vi "Midterm2.vi"() -> ()   [LabVIEW 2019]
uses:
  Program Files (x86)/National Instruments/LabVIEW 2019/project/EN1Course-master (12)/EN1Course-master/_Subs/ThingWorx/_TW_Subs/TW_XControl.xctl
  Program Files (x86)/National Instruments/LabVIEW 2019/project/EN1Course-master (12)/EN1Course-master/_Subs/ThingWorx/_TW_Subs/Thingworx_Write_string.vi
panel:
  in  "Date":string(xcontrol)="Day1:MadDATE"
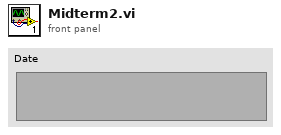
[diagram p1: front panel]
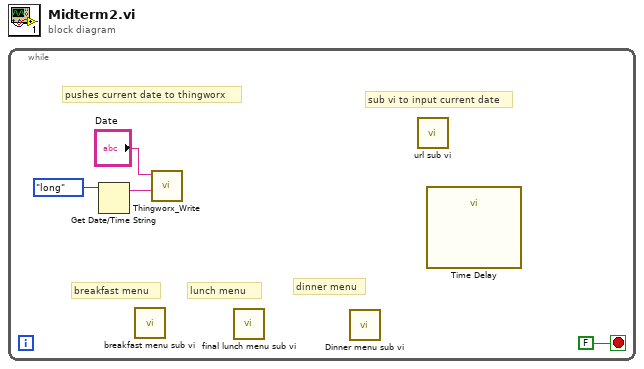
[diagram p0: block diagram]
diagram:
  n1 = while {
    stop <- FALSE stop-if-true
    # "dinner menu"
    # "lunch menu"
    # "breakfast menu"
    # "pushes current date to thingworx"
    # "sub vi to input current date"
    n2 = Get Date/Time String(date format (0)=enum16{"short", "long", "abbreviated"}."long") -> (date string=w4:string)  [unwired: 2 in, 1 out]
    n3 = call "breakfast menu sub vi.vi"() -> ()  [unwired: 12 in]
    n4 = call-poly "Thingworx_Write.vi"("String"=w4, "Thingworx"="Date") -> ()  [unwired: 10 in]
    n5 = call "final lunch menu sub vi.vi"() -> ()  [unwired: 12 in]
    n6 = call "Dinner menu sub vi.vi"() -> ()  [unwired: 12 in]
    n7 = call "url sub vi.vi"() -> ()  [unwired: 11 in, 1 out]
    n8 = call "Time Delay"() -> ()  [unwired: 11 in, 1 out]
  }
